vi "NACA0015.vi"() -> ()   [LabVIEW 2012]
uses:
  <vilib>/Utility/error.llb/DialogType.ctl
  <vilib>/Utility/file.llb/Read From Spreadsheet File (string).vi
  <vilib>/Analysis/baseanly.llb/Mean (DBL).vi
  <vilib>/Analysis/NI_AALBase.lvlib
panel:
  in  "Test Array_SS 2":dbl[](array[numeric])=[-10.0, -8.0, -6.0, -4.0, -2.0, 0.0, 2.0, 3.0, 4.0, 5.0, 6.0, 7.0, 8.0, 9.0, 10.0, 11.0, 12.0, 13.0, 14.0, 15.0, 16.0, 17.0, 18.0, 19.0, 20.0, 21.0, 0.0]
  in  "TS Temp (C)":dbl=27.0
  in  "Patm (inch Hg)":dbl=29.0
  out "Cm":cluster{"AOA_M":dbl, "AOA_Enc":dbl}(graph)
  out "U (m/s)":cluster{"AOA_M":dbl, "AOA_Enc":dbl}(graph)
  out "Cl":dbl(graph)
  out "AOA":cluster{"AOA_M":dbl, "AOA_Enc":dbl}(graph)={"AOA_M"=12.004225352112677, "AOA_Enc"=13.2}
  in  "next":bool
  out "Cp_rms":cluster{dbl[], dbl[]}[](graph)
  out "Cp_mean":cluster{dbl[], dbl[]}[](graph)
  in  "OK Button":bool
  in  "stop":bool
  in  "Incidence angles":i32(listbox)=17
  in  "Port map file":path=path "D:/Shreyas/Pressure_MEasurement/NACA0015_portmap1.txt"
  in  "Scanner #":i32=1
  in  "Model para":dbl[](array[numeric])=[310.0, 305.0] caption="Chord\n\nSpan"
  out "Current position (deg)":T1={"Axis 1"=14.4, "Axis 2"=13.005633802816902, "Axis 3"=0.0, "Axis 4"=0.0} {"Axis 4" format="%.3g"; "Axis 3" format="%.3g"; "Axis 2" format="%.3g"; "Axis 1" format="%.3g"}
  out "Uinf":dbl
  out "Qinf":dbl
  in  "Target position cluster":T2
  out "Pressure signal":dbl[][](graph)
  out "Exc":dbl=4.592317034403483 format="%.4f"
  in  "ESPdaq para":T3={"AI channels (ESP)"="PXI2Slot5/ai1:2,PXI2Slot5/ai0", "AI configuration"=10106, "DIO lines"="PXI2Slot5/port0/line0:7", "Counter Channel"="PXI2Slot5/ctr0", "Clock Source"="/PXI2Slot5/Ctr0InternalOutput", "Rate (Hz)"=16000.0, "duty cycle"=0.9} {"AI configuration" items=["default"=-1, "RSE"=10083, "NRSE"=10078, "Differential"=10106, "Pseudodifferential"=12529]; "duty cycle" format="%.6f"; "Rate (Hz)" format="%0.2f"}
  in  "Scanner coeff":T4
  in  "Espcal file":path=path "D:/Shreyas/ESP_cal_files/calcoefffinal"
  in  "Data record":T6={"Header"="", "Run para"=[], "Motion Para"={"Motion Board ID"=1, "Axis parameters in"=[{"Axis type"=1, " Velocity (rpm)"=4.0, " Acceln (rps\\s)"=1.0, " Deceln (rps\\s)"=1.0, "Enc Counts/Rev"=2880, "Kp"=30, "Kd"=800, "Td"=2}, {"Axis type"=2, " Velocity (rpm)"=4.0, " Acceln (rps\\s)"=1.0, " Deceln (rps\\s)"=1.0, "Enc Counts/Rev"=2880, "Kp"=30, "Kd"=800, "Td"=2}, {"Axis type"=0, " Velocity (rpm)"=4000.0, " Acceln (rps\\s)"=1000.0, " Deceln (rps\\s)"=1000.0, "Enc Counts/Rev"=8000, "Kp"=60, "Kd"=700, "Td"=5}, {"Axis type"=0, " Velocity (rpm)"=4000.0, " Acceln (rps\\s)"=1000.0, " Deceln (rps\\s)"=1000.0, "Enc Counts/Rev"=8000, "Kp"=60, "Kd"=700, "Td"=5}], "Axis status"={"Axis 1"=TRUE, "Axis 2"=TRUE, "Axis 3"=FALSE, "Axis 4"=FALSE, "Axis 5"=FALSE, "Axis 6"=FALSE, "Axis 7"=FALSE, "Axis 8"=FALSE}, "Current position"={"Axis 1"=0.0, "Axis 2"=0.0, "Axis 3"=0.0, "Axis 4"=0.0}}, "ESP DAQ para"={"AI channels (ESP)"="PXI1Slot7/ai0:4,PXI1Slot7/ai7", "AI configuration"=10106, "DIO lines"="PXI1Slot7/port0/line0:7", "Counter Channel"="PXI1Slot7/ctr0", "Clock Source"="/PXI1Slot7/Ctr0InternalOutput", "Rate (Hz)"=16000.0, "duty cycle"=0.9}, "Model para"=[], "Nowind data"=[], "Mean data"=[], "Port map_B19"=[], "ESP info"={"Cal header"="", "Calcoeff"=[]}, "rms data"=[]} {"ESP DAQ para"."AI configuration" items=["default"=-1, "RSE"=10083, "NRSE"=10078, "Differential"=10106, "Pseudodifferential"=12529]; "ESP DAQ para"."duty cycle" format="%.6f"; "ESP DAQ para"."Rate (Hz)" format="%0.2f"; "Motion Para"."Axis parameters in"."Axis type" items=["Free axis", "Master axis", "Slave axis"]; "Motion Para"."Axis parameters in"."Enc Counts/Rev" min=1; "Motion Para"."Axis parameters in"."Deceln (rps\\s)" max=2097152.0 step=1.0 format="%.2f"; "Motion Para"."Axis parameters in"."Acceln (rps\\s)" min=1.0 max=2097152.0 step=1.0 format="%.2f"; "Motion Para"."Axis parameters in"."Velocity (rpm)" min=-536870912.0 max=536870912.0 step=1.0 format="%.2f"; "Motion Para"."Axis parameters in"."Td" max=63; "Motion Para"."Axis parameters in"."Kd" max=32767; "Motion Para"."Axis parameters in"."Kp" max=32767; "Motion Para"."Motion Board ID" min=1 max=32 step=1}
  in  "Header":string="NACA 0015 Pressure Measurement for IR thermography, Shreyas Joshi, May 2016 "
  in  "Run Number":string="1"
  in  "Status":string="Initialization in progress"
  in  "start":bool
  # "Pressure measurement on NACA 0015 Airfoil"
  # "Input Parameters"
  # "Channel Parameters"
  # "Timing Parameters"
  # "Channel Parameters"
  # "Timing Parameters"
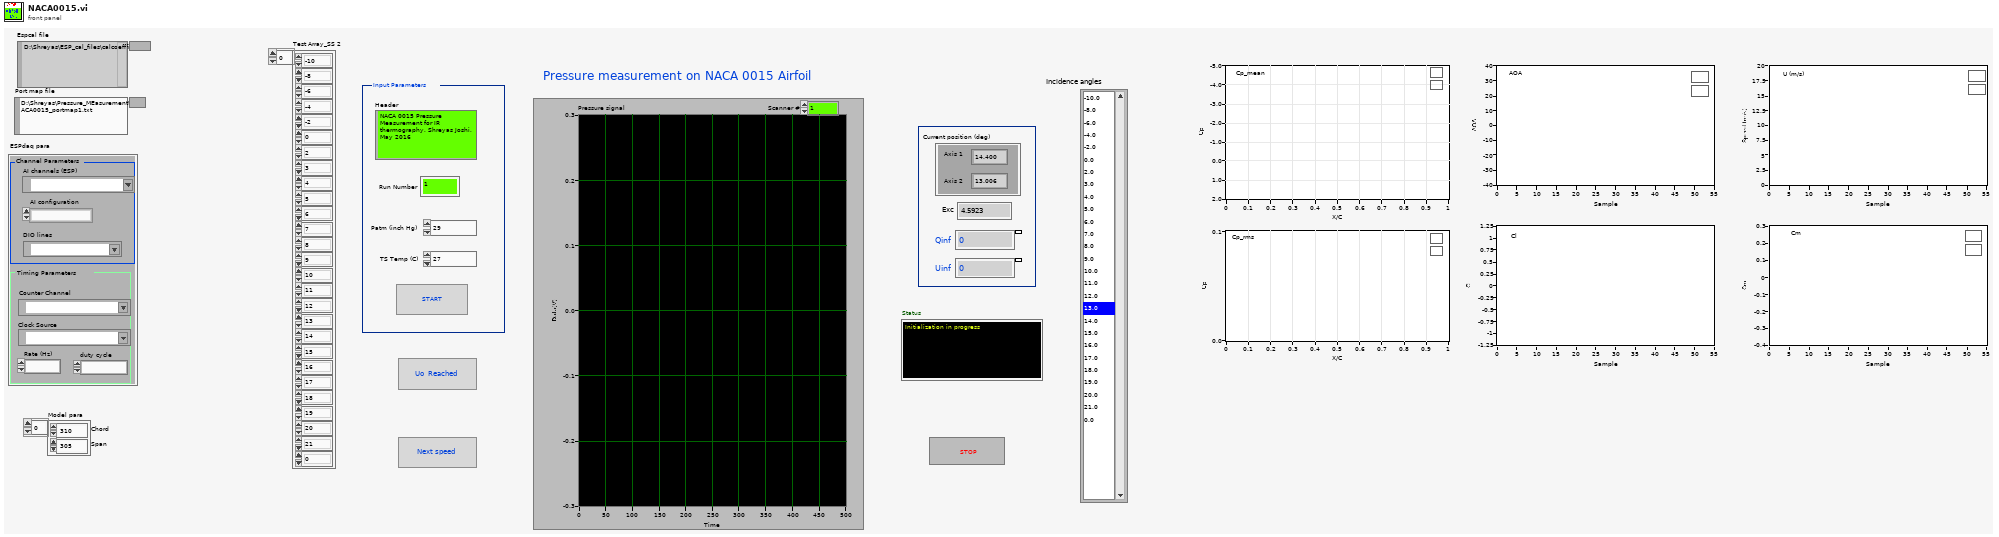
[diagram p1: front panel]
types:
  T1 = cluster{"Axis 1":dbl, "Axis 2":dbl, "Axis 3":dbl, "Axis 4":dbl}
  T2 = cluster{"Axis 1":i32, "Axis 2":i32, "Axis 3":i32, "Axis 4":i32}
  T3 = cluster{"AI channels (ESP)":tag, "AI configuration":i32, "DIO lines":tag, "Counter Channel":tag, "Clock Source":tag, "Rate (Hz)":dbl, "duty cycle":dbl}
  T4 = cluster{"ESP Cal header":string, "Scanner cal coefficients":dbl[][][]}
  T5 = typedef "Board Id" = u8
  T6 = cluster{"Header":string, "Run para":dbl[], "Motion Para":cluster{"Motion Board ID":T5, "Axis parameters in":cluster{"Axis type":u16, " Velocity (rpm)":dbl, " Acceln (rps\\s)":dbl, " Deceln (rps\\s)":dbl, "Enc Counts/Rev":u16, "Kp":u16, "Kd":u16, "Td":u16}[], "Axis status":cluster{"Axis 1":bool, "Axis 2":bool, "Axis 3":bool, "Axis 4":bool, "Axis 5":bool, "Axis 6":bool, "Axis 7":bool, "Axis 8":bool}, "Current position":cluster{"Axis 1":dbl, "Axis 2":dbl, "Axis 3":dbl, "Axis 4":dbl}}, "ESP DAQ para":cluster{"AI channels (ESP)":tag, "AI configuration":i32, "DIO lines":tag, "Counter Channel":tag, "Clock Source":tag, "Rate (Hz)":dbl, "duty cycle":dbl}, "Model para":dbl[], "Nowind data":dbl[][], "Mean data":dbl[][], "Port map_B19":string[][], "ESP info":cluster{"Cal header":string, "Calcoeff":dbl[][][]}, "rms data":dbl[][]}
  T7 = typedef "DialogType.ctl" = u16
  T8 = enum16{"open", "replace", "create", "open or create", "replace or create", "replace or create with confirmation"}
  T9 = cluster{"Motion Board ID":T5, "Axis parameters in":cluster{"Axis type":u16, " Velocity (rpm)":dbl, " Acceln (rps\\s)":dbl, " Deceln (rps\\s)":dbl, "Enc Counts/Rev":u16, "Kp":u16, "Kd":u16, "Td":u16}[], "Axis status":cluster{"Axis 1":bool, "Axis 2":bool, "Axis 3":bool, "Axis 4":bool, "Axis 5":bool, "Axis 6":bool, "Axis 7":bool, "Axis 8":bool}, "Current position":cluster{"Axis 1":dbl, "Axis 2":dbl, "Axis 3":dbl, "Axis 4":dbl}}
  T10 = cluster{"Ucc (m/s)":dbl, "AOA_m":dbl, "Cdp":dbl, "Cl":dbl, "Cmle":dbl, "Cmc/4":dbl, "Upp (m/s)":dbl, "AOA_Enc":dbl, "Qo (Pa)":dbl}
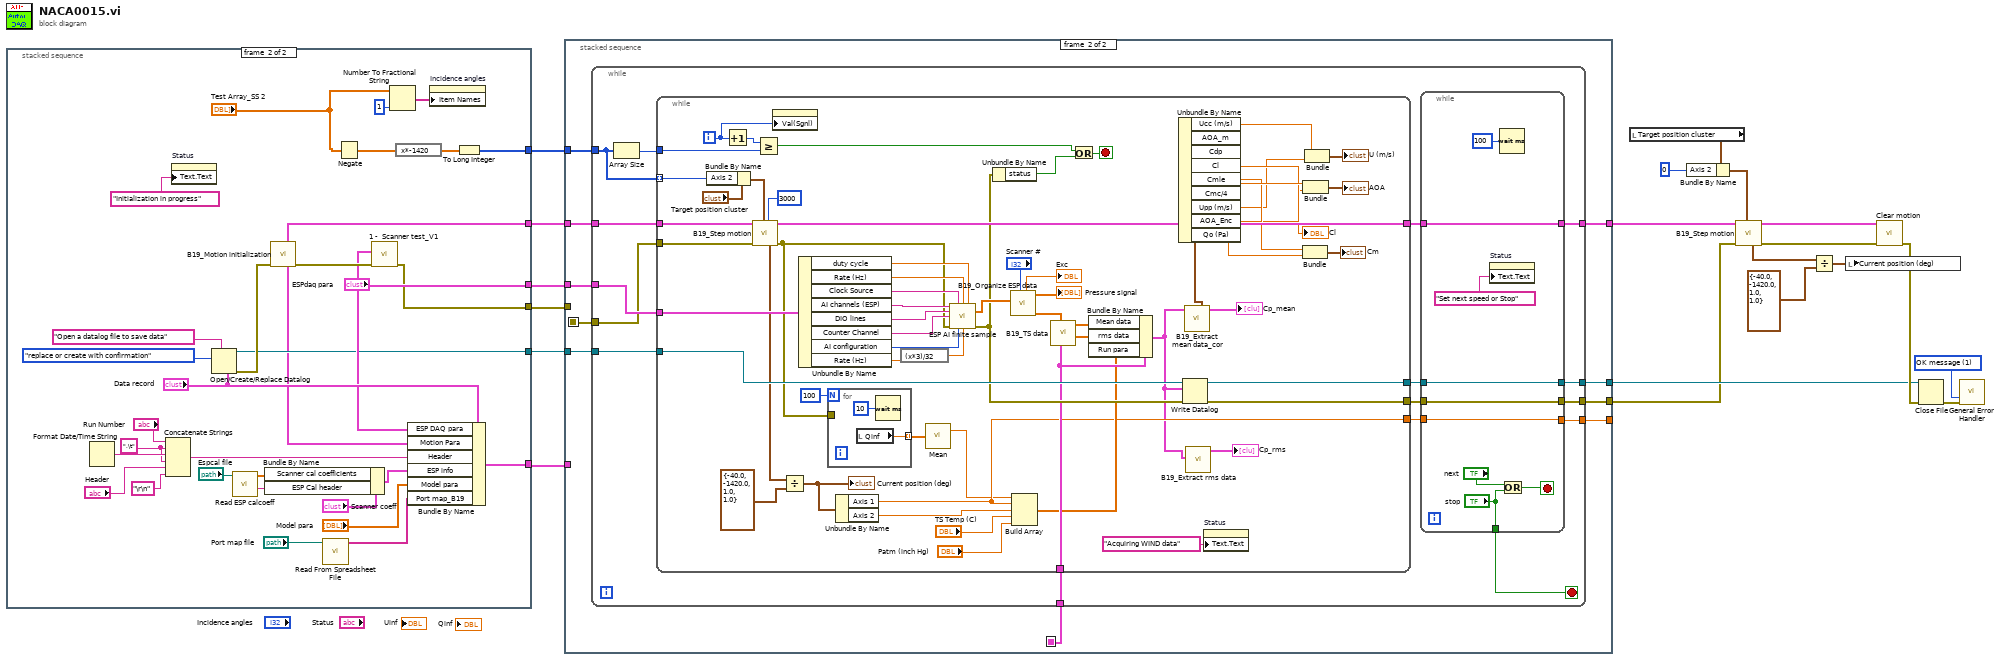
[diagram p0: block diagram]
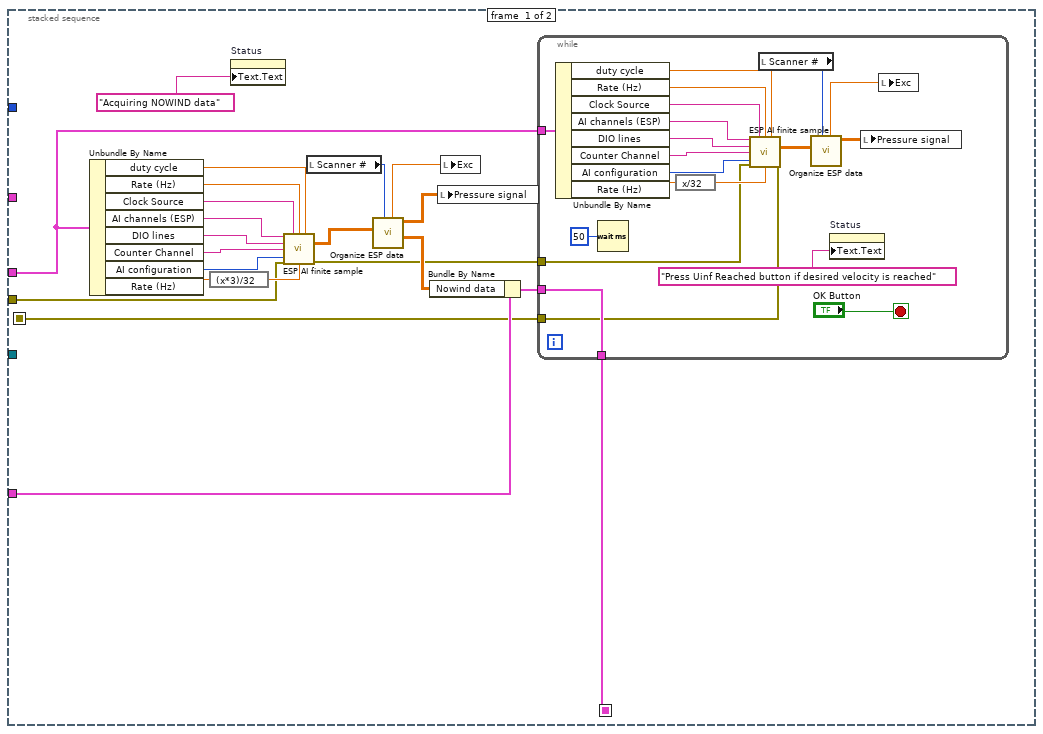
[diagram p2: hidden frame]
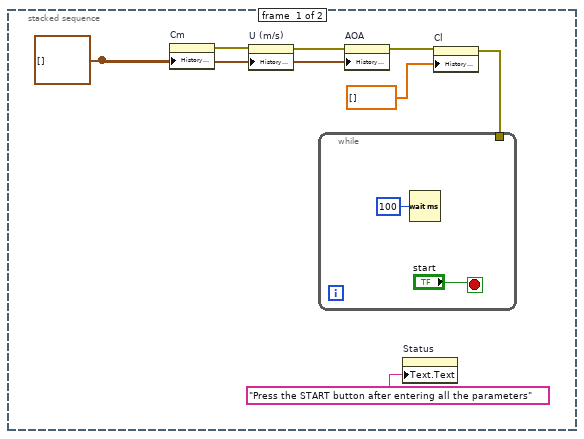
[diagram p3: hidden frame]
diagram:
  w13 = T7 1 items=["no dialog", "OK message", "continue or stop message", "OK message + warnings", "continue/stop + warnings"] ("type of dialog (OK msg:1)")
  n1 = stacked-sequence {
    tunnel: [_ w38] -> w16
    tunnel: [_ w39] -> w18
    tunnel: [_ "ESPdaq para"] -> w19
    tunnel: [_ w41] -> w20
    tunnel: [_ w40] -> w17
    tunnel: [_ w37] -> w15
    frame #0 {
      w26 = cluster{"AOA_M":dbl, "AOA_Enc":dbl}[] [] ("History Data")
      n2 = property on="Cm" class="WFChart (strict)"("History Data"=w26) -> (error out=w25:errorcluster)  [unwired: 2 in, 1 out]
      n3 = property on="U (m/s)" class="WFChart (strict)"(error in=w25, "History Data"=w26) -> (error out=w24:errorcluster)  [unwired: 1 in, 1 out]
      n4 = property on="AOA" class="WFChart (strict)"(error in=w24, "History Data"=w26) -> (error out=w23:errorcluster)  [unwired: 1 in, 1 out]
      n5 = property on="Status" class="Str"("Text.Text"="Press the START button after entering all the parameters") -> ()  [unwired: 2 in, 2 out]
      n6 = property on="Cl" class="WFChart (strict)"(error in=w23, "History Data"=dbl[] []) -> (error out=w22:errorcluster)  [unwired: 1 in, 1 out]
      n7 = while {
        tunnel: w22 -> [_]
        stop <- "start" stop-if-true
        n8 = Wait (ms)(milliseconds to wait=u32 100) -> ()  [unwired: 1 out]
      }
    }
    frame #1 {
      w58 = ",\t"
      n9 = Format Date/Time String() -> (date/time string=w59:string)  [unwired: 3 in]
      n10 = Concatenate Strings("Run Number", w58, w59, w58, "Header", "\r\n") -> (w46:string)
      n11 = property on="Status" class="Str"("Text.Text"="Initialization in progress") -> ()  [unwired: 2 in, 2 out]
      n12 = Open/Create/Replace Datalog ("New File")(5:"Data record", 7:"Open a datalog file to save data" ("prompt"), 10:T8."replace or create with confirmation" ("operation (0:open)")) -> (0:w48:errorcluster, 3:w38:refnum<k1>)  [unwired: 3 in, 1 out]
      n13 = call "Read ESP calcoeff.vi"("file path"="Espcal file") -> ("ESP Cal header"=w49:string, "Scanner cal coefficients"=w51:dbl[][][])  [unwired: 7 in]
      n14 = Bundle By Name(cluster="Scanner coeff", "Scanner cal coefficients"=w51, "ESP Cal header"=w49) -> (w45:T4)
      n15 = call "B19_Motion initialization.vi"("error in"=w48) -> ("error out"=w47:errorcluster, "Motion Parameters out"=w37:T9)  [unwired: 6 in, 1 out]
      n16 = call-poly <vilib>:"Read From Spreadsheet File.vi"("file path (dialog if empty)"="Port map file") -> ("all rows"=w32:string[][])  [unwired: 6 in, 4 out]
      n17 = Negate(x="Test Array_SS 2") -> (-x=w31:dbl[])
      n18 = call "1 -  Scanner test_V1.vi"("error in"=w47, "DAQ Parameters"="ESPdaq para") -> ("error out"=w39:errorcluster)  [unwired: 9 in]
      n19 = Number To Fractional String(number="Test Array_SS 2", precision (6)=i16 1) -> (F-format string=w33:string[])  [unwired: 2 in]
      n20 = expression code="x*-1420"(w31) -> (w42:dbl[])
      n21 = Bundle By Name(cluster="Data record", "ESP DAQ para"="ESPdaq para", "Motion Para"=w37, "Header"=w46, "ESP info"=w45, "Model para"="Model para", "Port map_B19"=w32) -> (w40:T6)
      n22 = property on="Incidence angles" class="LstBox (strict)"("Item Names"=w33) -> ()  [unwired: 2 in, 2 out]
      n23 = To Long Integer(number=w42) -> (32bit integer=w41:i32[])
    }
  }
  n24 = stacked-sequence {
    seq-local: [w61 _] -> [_ w106]
    seq-local: [w63 _] -> [_ w104]
    tunnel: w20 -> [_ w112]
    tunnel: w19 -> [w65 w110]
    tunnel: w18 -> [w72 _]
    tunnel: w17 -> [w70 _]
    tunnel: w16 -> [_ w105]
    tunnel: w15 -> [_ w111]
    tunnel: [_ w109] -> w11
    tunnel: [_ w108] -> w5
    tunnel: [_ w107] -> w10
    tunnel: [_ w103] -> _
    frame #0 {
      n25 = Unbundle By Name(w65) -> ("duty cycle"=w77:dbl, "Rate (Hz)"=w78:dbl, "Clock Source"=w79:tag, "AI channels (ESP)"=w81:tag, "DIO lines"=w80:tag, "Counter Channel"=w76:tag, "AI configuration"=w75:i32, "Rate (Hz)"=w74:dbl)
      n26 = expression code="(x*3)/32"(w74) -> (w73:dbl)
      n27 = property on="Status" class="Str"("Text.Text"="Acquiring NOWIND data") -> ()  [unwired: 2 in, 2 out]
      n28 = call "ESP AI finite sample.vi"("AI channels"=w81, "Clock Source"=w79, "Rate (Hz)"=w78, "duty cycle"=w77, "DIO lines"=w80, "Counter Channel"=w76, "error in"=w72, "AI terminal configuration"=w75, "Nsamples"=w73) -> ("Pressure data out"=w71:dbl[][], "error out"=w62:errorcluster)  [unwired: 5 in]
      n29 = local read "Scanner #"() -> (w66:i32)
      n30 = call "Organize ESP data.vi"("Scanner"=w66, "Data in"=w71) -> ("Normalized scanner data"=w69:dbl[][], "Raw data"=w67:dbl[][], "Exc"=w68:dbl)  [unwired: 5 in]
      n31 = Bundle By Name(cluster=w70, "Nowind data"=w69) -> (w64:T6)
      n32 = local write "Pressure signal"(w67) -> ()
      n33 = local write "Exc"(w68) -> ()
      n34 = while {
        tunnel: w65 -> [w90]
        tunnel: w64 -> [w88]
        tunnel: [w88] -> w63
        tunnel: w62 -> [w84]
        tunnel: [w83] -> w61
        stop <- "OK Button" stop-if-true
        n35 = Unbundle By Name(w90) -> ("duty cycle"=w95:dbl, "Rate (Hz)"=w94:dbl, "Clock Source"=w93:tag, "AI channels (ESP)"=w91:tag, "DIO lines"=w92:tag, "Counter Channel"=w96:tag, "AI configuration"=w97:i32, "Rate (Hz)"=w98:dbl)
        n36 = Wait (ms)(milliseconds to wait=u32 50) -> ()  [unwired: 1 out]
        n37 = expression code="x/32"(w98) -> (w89:dbl)
        n38 = call "ESP AI finite sample.vi"("AI channels"=w91, "Clock Source"=w93, "Rate (Hz)"=w94, "duty cycle"=w95, "DIO lines"=w92, "Counter Channel"=w96, "error in"=w84, "AI terminal configuration"=w97, "Nsamples"=w89) -> ("Pressure data out"=w99:dbl[][], "error out"=w83:errorcluster)  [unwired: 5 in]
        n39 = local read "Scanner #"() -> (w102:i32)
        n40 = call "Organize ESP data.vi"("Scanner"=w102, "Data in"=w99) -> ("Raw data"=w101:dbl[][], "Exc"=w100:dbl)  [unwired: 5 in, 1 out]
        n41 = property on="Status" class="Str"("Text.Text"="Press Uinf Reached button if desired velocity is reached") -> ()  [unwired: 2 in, 2 out]
        n42 = local write "Pressure signal"(w101) -> ()
        n43 = local write "Exc"(w100) -> ()
      }
    }
    frame #1 {
      n44 = while {
        tunnel: w112 -> [w127]
        tunnel: w111 -> [w126]
        tunnel: w110 -> [w125]
        tunnel: [w118] -> w109
        tunnel: [w116] -> w108
        tunnel: [w120] -> w107
        tunnel: w106 -> [w124]
        tunnel: w105 -> [w123]
        tunnel: w104 -> [w122]
        tunnel: [w113] -> w103
        stop <- w115 stop-if-true
        n45 = Array Size(array=w127) -> (size(s)=w128:i32)
        n46 = while {
          tunnel: w128 -> [w196]
          tunnel: w127 -> [w197] mode=indexing
          tunnel: w126 -> [w195]
          tunnel: w124 -> [w194]
          tunnel: w125 -> [w184]
          tunnel: w122 -> [w167]
          tunnel: [w181] -> w119
          tunnel: [w180] -> w117
          tunnel: [w179] -> w121
          tunnel: w123 -> [w176]
          tunnel: [w158] -> w114
          i -> [w171]
          stop <- w183 stop-if-true
          n47 = Bundle By Name(cluster="Target position cluster", "Axis 2"=w197) -> (w193:T2)
          n48 = Increment(x=w171) -> (x+1=w198:i32)
          n49 = call "B19_Step motion.vi"("wait after motion (ms)"=u32 3000, "Target position (counts)"=w193, "error in"=w194, "Motion Parameters"=w195) -> ("Error out"=w157:errorcluster, "Motion Parameters out"=w179:T9, "Current position (counts)"=w160:T2)  [unwired: 5 in]
          n50 = Greater Or Equal?(x=w198, y=w196) -> (x >= y?=w182:bool)
          n51 = property on="Incidence angles" class="LstBox (strict)"("Val(Sgnl)"=w171) -> ()  [unwired: 2 in, 2 out]
          n52 = Divide(x=w160, y=T1 {"Axis 1"=-40.0, "Axis 2"=-1420.0, "Axis 3"=1.0, "Axis 4"=1.0}) -> (x/y=w163:T1)
          "Current position (deg)" <- w163
          n53 = Unbundle By Name(w184) -> ("duty cycle"=w187:dbl, "Rate (Hz)"=w188:dbl, "Clock Source"=w189:tag, "AI channels (ESP)"=w191:tag, "DIO lines"=w190:tag, "Counter Channel"=w186:tag, "AI configuration"=w185:i32, "Rate (Hz)"=w178:dbl)
          n54 = for {
            N: 100 -> [_]
            tunnel: w157 -> [_]
            tunnel: [w200] -> w155 mode=indexing
            n55 = local read "Qinf"() -> (w200:dbl)
            n56 = Wait (ms)(milliseconds to wait=u32 10) -> ()  [unwired: 1 out]
          }
          n57 = Unbundle By Name(w163) -> ("Axis 1"=w158:dbl, "Axis 2"=w159:dbl)
          n58 = expression code="(x*3)/32"(w178) -> (w177:dbl)
          n59 = call-poly <vilib>:"Mean.vi"("X"=w155) -> ("mean"=w154:dbl)  [unwired: 1 out]
          n60 = call "ESP AI finite sample.vi"("AI channels"=w191, "Clock Source"=w189, "Rate (Hz)"=w188, "duty cycle"=w187, "DIO lines"=w190, "Counter Channel"=w186, "error in"=w157, "AI terminal configuration"=w185, "Nsamples"=w177) -> ("Pressure data out"=w175:dbl[][], "error out"=w169:errorcluster)  [unwired: 5 in]
          n61 = Unbundle By Name(w169) -> ("status"=w162:bool)
          n62 = call "B19_Organize ESP data.vi"("Scanner"="Scanner #", "Data in"=w175) -> ("ESP data (V/Vexc)"=w168:dbl[][][], "ESP data (V)"=→"Pressure signal":dbl[][], "Exc"=→"Exc":dbl)  [unwired: 5 in]
          n63 = Build Array(w154, w158, w159, "TS Temp (C)", "Patm (inch Hg)") -> (w166:dbl[])
          n64 = call "B19_TS data.vi"("Data record"=w167, "ESP: wind data"=w168) -> ("rms data"=w164:dbl[][], "Mean data"=w165:dbl[][])  [unwired: 8 in]
          n65 = Or(x=w182, y=w162) -> (x .or. y?=w183:bool)
          n66 = Bundle By Name(cluster=w167, "Mean data"=w165, "rms data"=w164, "Run para"=w166) -> (w138:T6)
          n67 = Write Datalog(4:w169, 6:w138, 7:w176) -> (0:w180:errorcluster, 3:w181:refnum<k1>)
          n68 = call "B19_Extract mean data_cor.vi"("Data record"=w138) -> ("Main Cp_mean"=→"Cp_mean":cluster{"XL/C":dbl[], "Cpl":dbl[]}[], "Airfoil characteristics"=w149:T10)  [unwired: 6 in, 1 out]
          n69 = Unbundle By Name(w149) -> ("Ucc (m/s)"=w148:dbl, "AOA_m"=w147:dbl, "Cl"=→"Cl":dbl, "Cmle"=w145:dbl, "Cmc/4"=w144:dbl, "Upp (m/s)"=w143:dbl, "AOA_Enc"=w142:dbl)  [unwired: 2 out]
          n70 = call "B19_Extract rms data.vi"("Data record"=w138) -> ("Cp_rms"=→"Cp_rms":cluster{"XL/C":dbl[], "Cpl":dbl[]}[])  [unwired: 6 in, 2 out]
          n71 = property on="Status" class="Str"("Text.Text"="Acquiring WIND data") -> ()  [unwired: 2 in, 2 out]
          n72 = Bundle("Cmle"=w145, "Cmc/4"=w144) -> (→"Cm":cluster{"Cmle":dbl, "Cmc/4":dbl})  [unwired: 1 in]
          n73 = Bundle("AOA_m"=w147, "AOA_Enc"=w142) -> (→"AOA":cluster{"AOA_m":dbl, "AOA_Enc":dbl})  [unwired: 1 in]
          n74 = Bundle("Ucc (m/s)"=w148, "Upp (m/s)"=w143) -> (→"U (m/s)":cluster{"Ucc (m/s)":dbl, "Upp (m/s)":dbl})  [unwired: 1 in]
        }
        n75 = while {
          tunnel: [w137] -> w120
          tunnel: w121 -> [w137]
          tunnel: w119 -> [w136]
          tunnel: [w136] -> w118
          tunnel: w117 -> [w135]
          tunnel: [w135] -> w116
          tunnel: ["stop"] -> w115
          tunnel: [w129] -> w113
          tunnel: w114 -> [w129]
          stop <- w133 stop-if-true
          n76 = property on="Status" class="Str"("Text.Text"="Set next speed or Stop") -> ()  [unwired: 2 in, 2 out]
          n77 = Wait (ms)(milliseconds to wait=u32 100) -> ()  [unwired: 1 out]
          n78 = Or(x="next", y="stop") -> (x .or. y?=w133:bool)
        }
      }
    }
  }
  n79 = local read "Target position cluster"() -> (w8:T2)
  n80 = Bundle By Name(cluster=w8, "Axis 2"=0) -> (w7:T2)
  n81 = call "B19_Step motion.vi"("Target position (counts)"=w7, "error in"=w5, "Motion Parameters"=w10) -> ("Error out"=w6:errorcluster, "Motion Parameters out"=w9:T9, "Current position (counts)"=w4:T2)  [unwired: 6 in]
  n82 = Divide(x=w4, y=T1 {"Axis 1"=-40.0, "Axis 2"=-1420.0, "Axis 3"=1.0, "Axis 4"=1.0}) -> (x/y=w3:T1)
  n83 = local write "Current position (deg)"(w3) -> ()
  n84 = call "Clear motion.vi"("error in"=w6, "Motion Parameters"=w9) -> ("error out"=w12:errorcluster)  [unwired: 6 in, 1 out]
  n85 = Close File(refnum=w11, error in=w12) -> (error out=w14:errorcluster)  [unwired: 1 out]
  n86 = call <vilib>:"General Error Handler.vi"("type of dialog (OK msg:1)"=w13, "error in (no error)"=w14) -> ()  [unwired: 9 in, 5 out]
